vi "Set - Elevator Status.vi"(8 "error in (no error)":errorcluster, 10 "Elevator Status":T1, 11 "View Model":T2) -> (0 "error out":errorcluster, 3 "View Model":T2)   [LabVIEW 2017]
doc: "Set actual value of Elevator Status to DVR."
uses:
  Controls/View Model.ctl
  Controls/Shared Model.ctl
  Error Handler/Controls/Error Model.ctl
  Error Handler/Controls/Error Data.ctl
  Error Handler/Controls/Error Level.ctl
  Configuration/Controls/Config Model.ctl
  Configuration/Controls/Config Data Record.ctl
  Configuration/Controls/Config Command.ctl
  Controller/Controls/Control Model.ctl
  Controller/Controls/Elevator Location.ctl
  Controller/Controls/Elevator Status.ctl
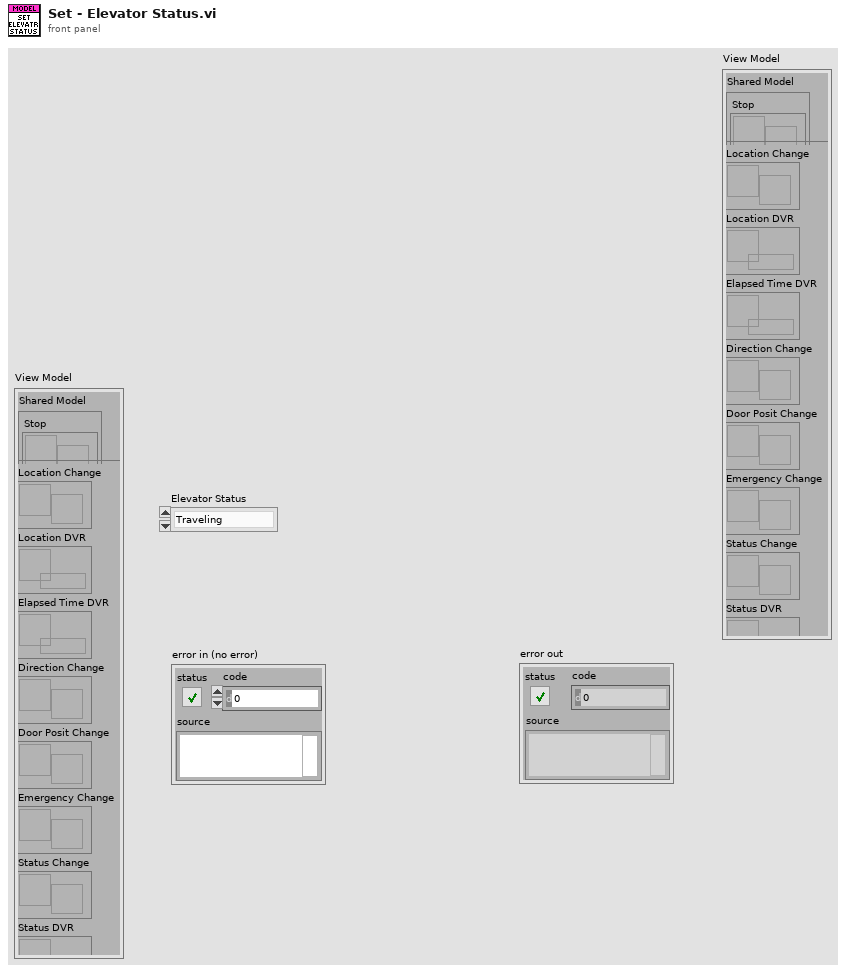
[diagram p1: front panel]
types:
  T1 = typedef "Elevator Status.ctl" = enum16{"Traveling", "Final Stop", "Medium Stop", "Idle"}
  T2 = typedef "View Model.ctl" = cluster{"Shared Model":T3, "Error Model":T4, "Config Model":T5, "Control Model":T6}
  T3 = typedef "Shared Model.ctl" = cluster{"Stop":refnum<user-event>, "Stop DVR":refnum<data-value>}
  T4 = typedef "Error Model.ctl" = cluster{"Error":refnum<user-event>}
  T5 = typedef "Config Model.ctl" = cluster{"Data DVR":refnum<data-value>, "Config CMD":refnum<user-event>}
  T6 = typedef "Control Model.ctl" = cluster{"Location Change":refnum<user-event>, "Location DVR":refnum<data-value>, "Elapsed Time DVR":refnum<data-value>, "Direction Change":refnum<user-event>, "Door Posit Change":refnum<user-event>, "Emergency Change":refnum<user-event>, "Status Change":refnum<user-event>, "Status DVR":refnum<data-value>}
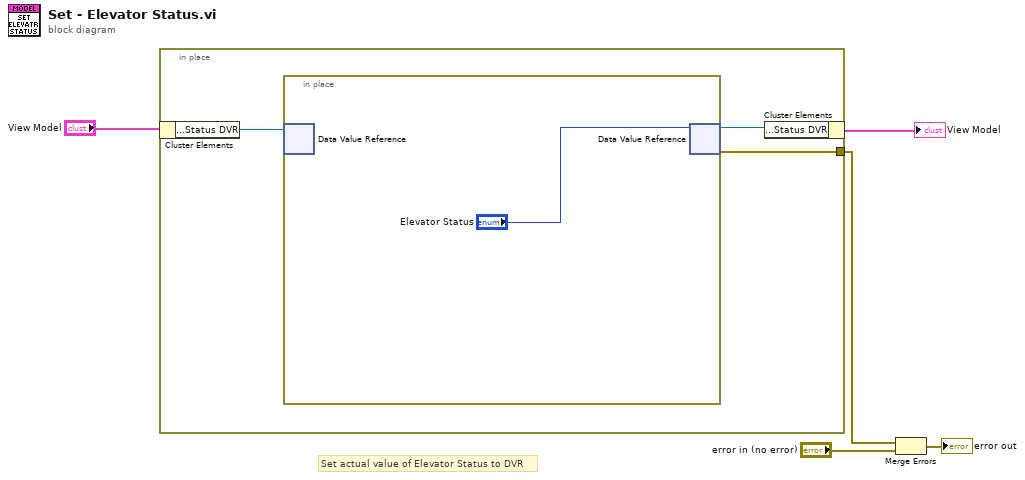
[diagram p0: block diagram]
diagram:
  # "Set actual value of Elevator Status to DVR"
  n1 = in-place {
    in-place-border: [w6] -> w3
    n2 = in-place-cluster #1("View Model") -> ("Control Model.Status DVR"=w8:refnum<data-value>)
    n3 = in-place {
      n4 = in-place-dvr #2(w8) -> ()  [unwired: 2 out]
      n5 = in-place-dvr #2("Elevator Status") -> (w7:refnum<data-value>, w6:errorcluster)
    }
    n6 = in-place-cluster #1("Control Model.Status DVR"=w7) -> (→"View Model":T2)
  }
  n7 = Merge Errors(w3, "error in (no error)") -> (→"error out":errorcluster)
